vi "Edit Config.vi"(8 "error in (no error)":errorcluster, 11 "General Parser in":refnum<class "General Parser.lvclass">) -> (0 "error out":errorcluster, 3 "General Parser out":refnum<class "General Parser.lvclass">)   [LabVIEW 2024, in "General Parser.lvclass"]
doc: "General Parser.lvclass:Edit Config.vi\n\nThis VI is used to edit the General Parser configuration parameters.\n\nInstrument Communication Module Version 1.0\nSeptember, 2017 Original Code Consulting David Thomson\n www.originalcode.com"
uses:
  General Parser.lvclass
  General Parser Config.ctl
  ICM Class Editor State.ctl
  ICM Editor Command.ctl
  General Parser.lvclass/General Parser.ctl
  Inside MICAS-X Global.vi
panel:
  in  "Import":bool
  in  "Test":bool
  in  "Flash Save":bool
  in  "Save":bool
  in  "Revert":bool
  in  "General Parse Config":T1
  # "The General Parser can be used to parse many data\nstrings using a standard LabVIEW format string. ICM\nalso includes additional formatting functions that are\ndescribed in the documentation."
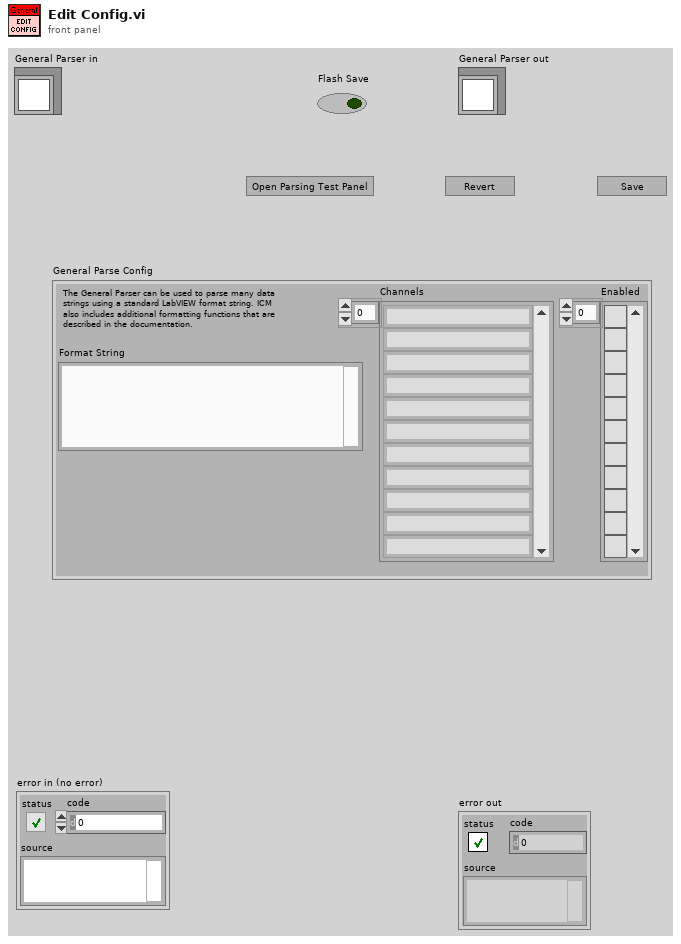
[diagram p1: front panel]
types:
  T1 = typedef "General Parser.lvclass/General Parser Config.ctl" = cluster{"Format String":string, "Channels":string[], "Enabled":bool[]}
  T2 = typedef "ICM Editor Command.ctl" = enum16{"No-op", "Exit"}
  T3 = typedef "ICM Class Editor State.ctl" = enum16{"Init", "Wait", "Write", "Read", "Display", "Set Flashing", "Error", "Stop"}
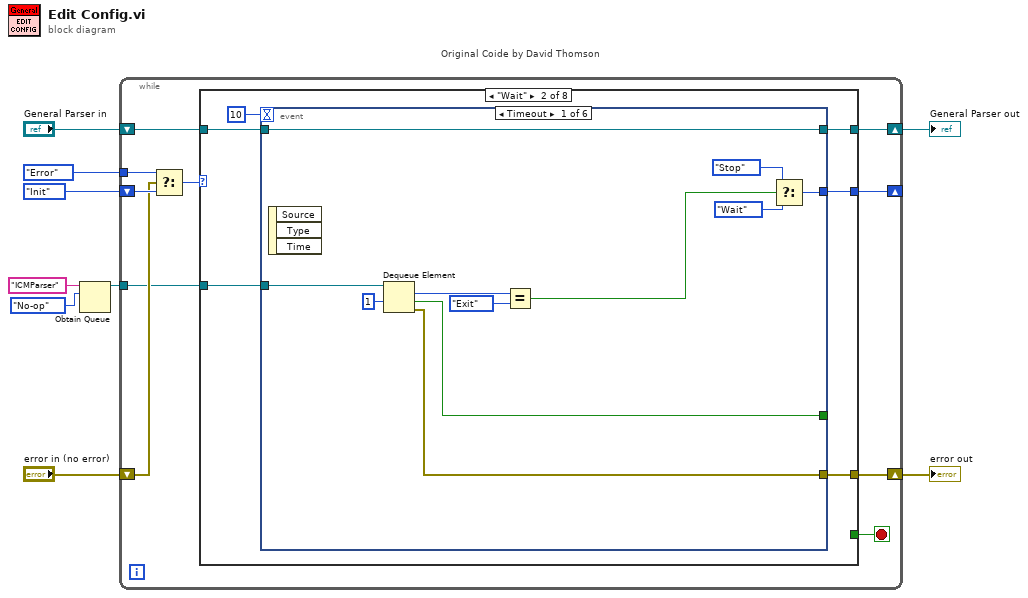
[diagram p0: block diagram]
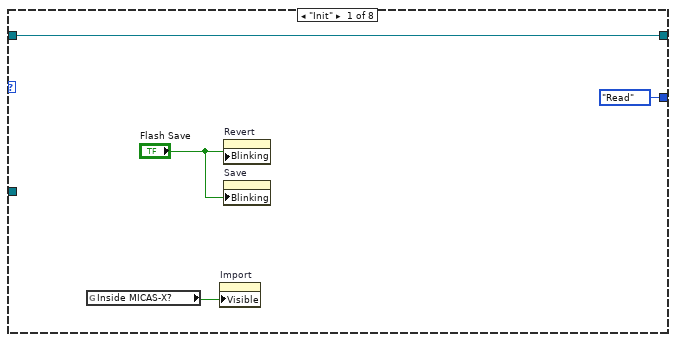
[diagram p2: hidden frame]
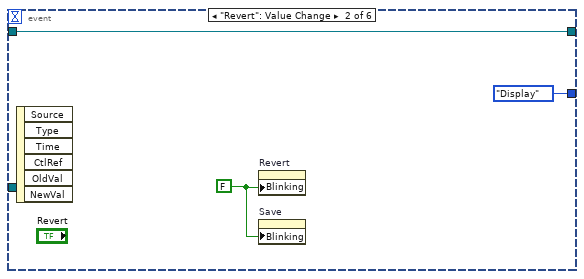
[diagram p3: hidden frame]
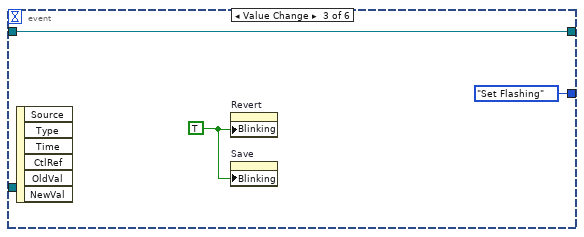
[diagram p4: hidden frame]
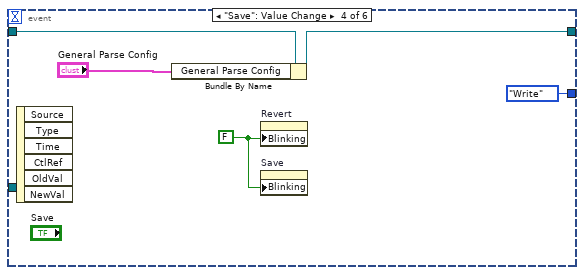
[diagram p5: hidden frame]
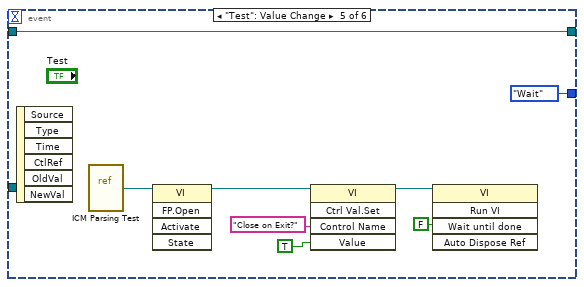
[diagram p6: hidden frame]
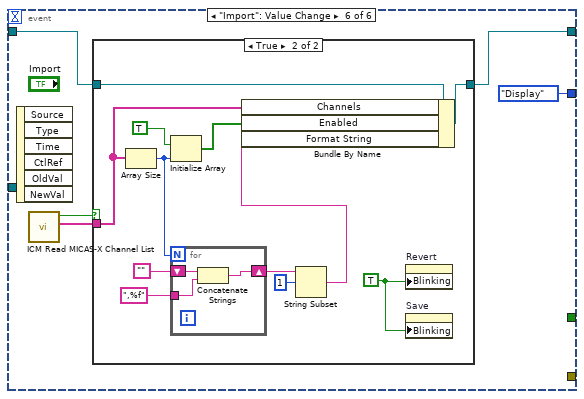
[diagram p7: hidden frame]
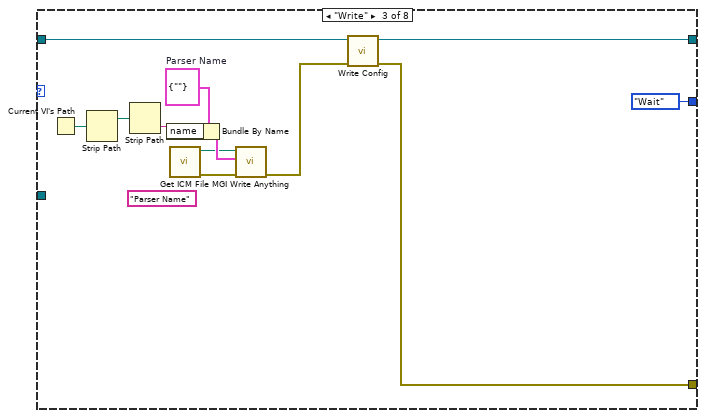
[diagram p9: hidden frame]
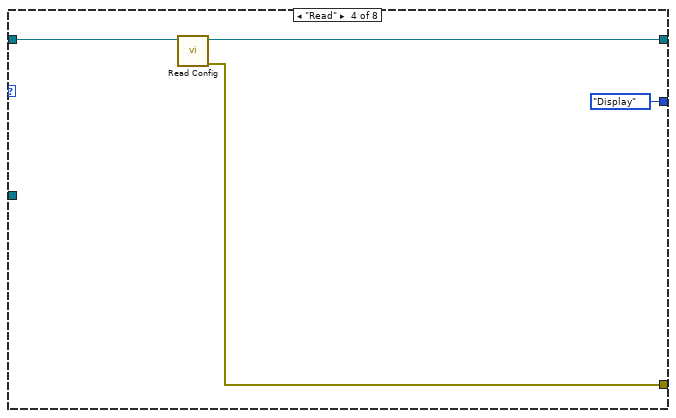
[diagram p10: hidden frame]
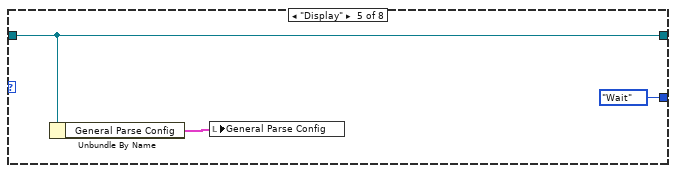
[diagram p11: hidden frame]
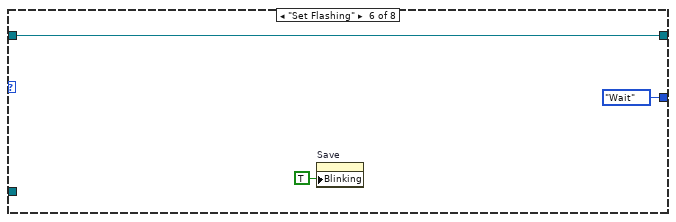
[diagram p12: hidden frame]
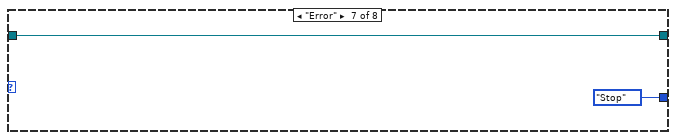
[diagram p13: hidden frame]
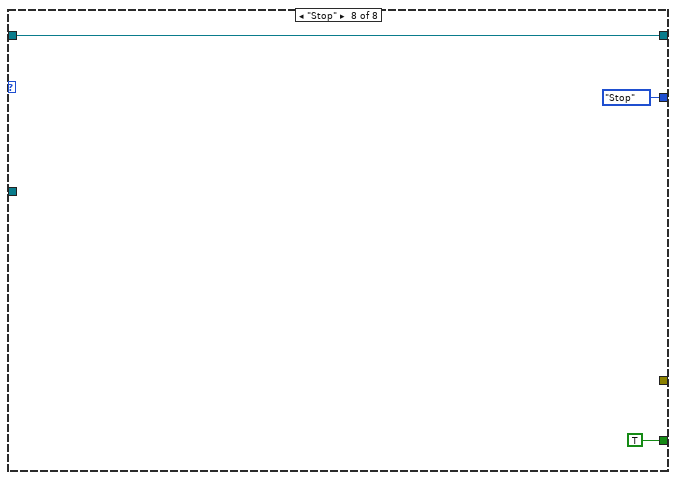
[diagram p14: hidden frame]
diagram:
  n1 = Obtain Queue(name (unnamed)="ICMParser", element data type=ICM_Editor_Command."No-op" ("Editor Command")) -> (queue out=w1:refnum<queue>)  [unwired: 3 in, 2 out]
  n2 = while "Original Coide by David Thomson" {
    shift-right: [w19] -> w8
    shift-left: "General Parser in" -> [w18]
    shift-right: [w12] -> _
    shift-left: ICM_Class_Editor_State."Init" ("Config State") -> [w16]
    shift-right: [w11] -> w6
    shift-left: "error in (no error)" -> [w14]
    tunnel: ICM_Class_Editor_State."Error" ("Config State") -> [w13]
    tunnel: w1 -> [w10]
    stop <- w17 stop-if-true
    n3 = Select(t=w13, s=w14, f=w16) -> (s? t:f=w15:T3)
    n4 = case shown="\"Wait\"" w15 {
      tunnel: [w22 w27 w90 w94 w99 w102 w104 w107] -> w19
      tunnel: w18 -> [w22 w26 w91 w96 w99 w102 w104 w107]
      tunnel: [_ _ _ _ _ _ _ TRUE] -> w17
      tunnel: [ICM_Class_Editor_State."Read" ("Config State") w28 ICM_Class_Editor_State."Wait" ("Config State") ICM_Class_Editor_State."Display" ("Config State") ICM_Class_Editor_State."Wait" ("Config State") ICM_Class_Editor_State."Wait" ("Config State") ICM_Class_Editor_State."Stop" ("Config State") ICM_Class_Editor_State."Stop" ("Config State")] -> w12
      tunnel: [_ w24 w89 w95 _ _ _ _] -> w11
      tunnel: w10 -> [_ w25 _ _ _ _ _ _]
      frame "Init" {
        n5 = global read "Inside MICAS-X Global.vi" "Inside MICAS-X?"() -> (w20:bool)
        n6 = property on="Import" class="Bool"("Visible"=w20) -> ()  [unwired: 2 in, 2 out]
        n7 = property on="Revert" class="Bool"("Blinking"="Flash Save") -> ()  [unwired: 2 in, 2 out]
        n8 = property on="Save" class="Bool"("Blinking"="Flash Save") -> ()  [unwired: 2 in, 2 out]
      }
      frame "Wait" {
        n9 = event shown="[0] Timeout" {
          selector: _ -> [_ _ _ _ _ _]
          dyn-events: _ -> [_ _ _ _ _ _]
          timeout: 10 -> [_ _ _ _ _ _]
          tunnel: [w37 ICM_Class_Editor_State."Display" ("Config State") ICM_Class_Editor_State."Set Flashing" ("Config State") ICM_Class_Editor_State."Write" ("Config State") ICM_Class_Editor_State."Wait" ("Config State") ICM_Class_Editor_State."Display" ("Config State")] -> w28
          tunnel: [w40 w42 w46 w48 w59 w61] -> w27
          tunnel: w26 -> [w40 w42 w46 w49 w59 w62]
          tunnel: w25 -> [w39 _ _ _ _ _]
          tunnel: [w31 _ _ _ _ _] -> w24
          tunnel: [w30 _ _ _ _ _] -> _
          event Timeout {
            n10 = event-data() -> ()  [unwired: 1 in, 3 out]
            n11 = Dequeue Element(queue=w39, timeout in ms (-1)=1) -> (element=w36:T2, timed out?=w30:bool, error out=w31:errorcluster)  [unwired: 1 in, 1 out]
            n12 = Equal?(x=w36, y=ICM_Editor_Command."Exit") -> (x = y?=w34:bool)
            n13 = Select(t=ICM_Class_Editor_State."Stop" ("Config State"), s=w34, f=ICM_Class_Editor_State."Wait" ("Config State")) -> (s? t:f=w37:T3)
          }
          event "Revert": Value Change {
            w41 = FALSE ("Blinking")
            n14 = event-data() -> ()  [unwired: 1 in, 6 out]
            n15 = property on="Revert" class="Bool"("Blinking"=w41) -> ()  [unwired: 2 in, 2 out]
            n16 = property on="Save" class="Bool"("Blinking"=w41) -> ()  [unwired: 2 in, 2 out]
          }
          event Value Change {
            w44 = TRUE ("Blinking")
            n17 = event-data() -> ()  [unwired: 1 in, 6 out]
            n18 = property on="Revert" class="Bool"("Blinking"=w44) -> ()  [unwired: 2 in, 2 out]
            n19 = property on="Save" class="Bool"("Blinking"=w44) -> ()  [unwired: 2 in, 2 out]
          }
          event "Save": Value Change {
            w47 = FALSE ("Blinking")
            n20 = event-data() -> ()  [unwired: 1 in, 6 out]
            n21 = Bundle By Name(cluster=w49, "General Parse Config"="General Parse Config") -> (w48:refnum<class "General Parser.lvclass">)
            n22 = property on="Revert" class="Bool"("Blinking"=w47) -> ()  [unwired: 2 in, 2 out]
            n23 = property on="Save" class="Bool"("Blinking"=w47) -> ()  [unwired: 2 in, 2 out]
          }
          event "Test": Value Change {
            n24 = event-data() -> ()  [unwired: 1 in, 6 out]
            n25 = vi-ref "ICM Parsing Test.vi"() -> (w57:refnum<vi>)
            n26 = invoke class="VI" method="FP.Open"(reference=w57) -> (reference out=w55:refnum<vi>)  [unwired: 4 in, 4 out]
            n27 = invoke class="VI" method="Ctrl Val.Set"(reference=w55, "Control Name"="Close on Exit?", "Value"=TRUE) -> (reference out=w54:refnum<vi>)  [unwired: 2 in, 4 out]
            n28 = invoke class="VI" method="Run VI"(reference=w54, "Wait until done"=FALSE ("Wait Until Done")) -> ()  [unwired: 3 in, 5 out]
          }
          event "Import": Value Change {
            n29 = event-data() -> ()  [unwired: 1 in, 6 out]
            n30 = call "ICM Read MICAS-X Channel List.vi"() -> ("Channels"=w60:string[], "Import?"=w63:bool)  [unwired: 10 in]
            n31 = case shown="True" w63 {
              tunnel: w62 -> [w65 w77]
              tunnel: [w65 w76] -> w61
              tunnel: w60 -> [_ w75]
              frame False {
              }
              frame True {
                w66 = TRUE ("Blinking")
                n32 = Array Size(array=w75) -> (size(s)=w72:i32)
                n33 = Initialize Array(TRUE, w72) -> (w73:bool[])
                n34 = for {
                  N: w72 -> [_]
                  shift-right: [w78] -> w69
                  shift-left: "" -> [w80]
                  tunnel: ",%f" -> [w79]
                  n35 = Concatenate Strings(w80, w79) -> (w78:string)
                }
                n36 = String Subset(string=w69, offset (0)=1) -> (substring=w67:string)  [unwired: 1 in]
                n37 = Bundle By Name(cluster=w77, "Channels"=w75, "Enabled"=w73, "Format String"=w67) -> (w76:refnum<class "General Parser.lvclass">)
                n38 = property on="Revert" class="Bool"("Blinking"=w66) -> ()  [unwired: 2 in, 2 out]
                n39 = property on="Save" class="Bool"("Blinking"=w66) -> ()  [unwired: 2 in, 2 out]
              }
            }
          }
        }
      }
      frame "Write" {
        w83 = cluster{"name":string} {"name"=""}  # Parser Name
        (unwired) "Parser Name" ("Section Name (Name of \"Anything\")")
        n40 = Current VI's Path() -> (path=w88:path)
        n41 = Strip Path(path=w88) -> (stripped path=w87:path)  [unwired: 1 out]
        n42 = Strip Path(path=w87) -> (name=w84:string)  [unwired: 1 out]
        n43 = Bundle By Name(cluster=w83, "name"=w84) -> (w85:cluster{"name":string})
        n44 = call "Get ICM File.vi"() -> ("error out"=w86:errorcluster, "ICM File"=w81:path)  [unwired: 10 in]
        n45 = call "MGI Write Anything.vi"("Error In"=w86, "Anything"=w85, "Path (dialog)"=w81) -> ("Error Out"=w82:errorcluster)  [unwired: 6 in, 2 out]
        n46 = call-dynamic "Write Config.vi"("error in (no error)"=w82, "General Parser in"=w91) -> ("error out"=w89:errorcluster, "General Parser out"=w90:refnum<class "General Parser.lvclass">)  [unwired: 8 in]
      }
      frame "Read" {
        n47 = call-dynamic "Read Config.vi"("General Parser in"=w96) -> ("error out"=w95:errorcluster, "General Parser out"=w94:refnum<class "General Parser.lvclass">)  [unwired: 9 in]
      }
      frame "Display" {
        n48 = Unbundle By Name(w99) -> ("General Parse Config"=w98:T1)
        n49 = local write "General Parse Config"(w98) -> ()
      }
      frame "Set Flashing" {
        n50 = property on="Save" class="Bool"("Blinking"=TRUE) -> ()  [unwired: 2 in, 2 out]
      }
      frame "Error" {
      }
      frame "Stop" {
      }
    }
  }
  "error out" <- w6
  "General Parser out" <- w8
